vi "interface.vi"(8 "error in (no error)":errorcluster, 10 "TCP Network Connection Refnum":refnum<k5>) -> (0 "error out":errorcluster, 2 "String":string, 3 "Error Code":i32)   [LabVIEW 2017]
doc: "Reads from TCP and parses into a return string. The first four bytes of the TCP string are the error code, the next four are the length of the message. These are converted to integers and formatted at the begining of the message."
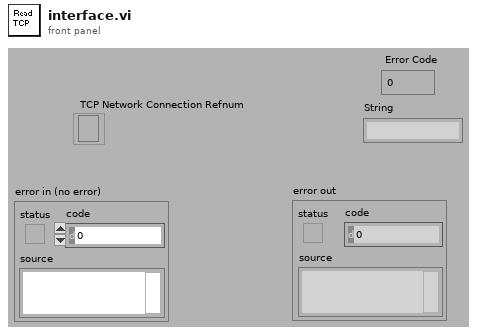
[diagram p1: front panel]
types:
  T1 = enum16{"Standard", "Buffered", "CRLF", "Immediate"}
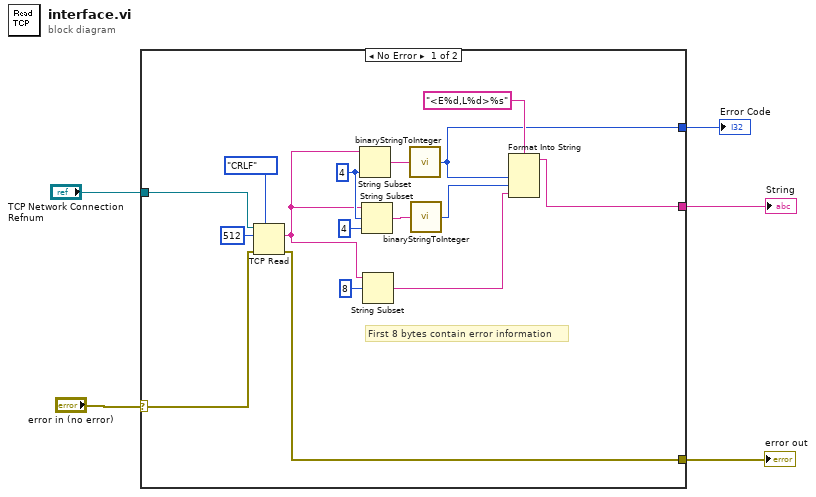
[diagram p0: block diagram]
diagram:
  n1 = case shown="No Error" "error in (no error)" {
    selector: "error in (no error)" -> [w18 w22]
    tunnel: [w17 w22] -> w4
    tunnel: [w10 _] -> w3
    tunnel: "TCP Network Connection Refnum" -> [w20 _]
    tunnel: [w6 _] -> w1
    frame No Error {
      w15 = 4 ("length (rest)")
      # "First 8 bytes contain error information"
      n2 = TCP Read(connection ID=w20, bytes to read=512, error in (no error)=w18, 7:T1."CRLF" ("mode (standard)")) -> (data out=w13:string, error out=w17:errorcluster)  [unwired: 1 in, 1 out]
      n3 = String Subset(string=w13, length (rest)=w15) -> (substring=w8:string)  [unwired: 1 in]
      n4 = String Subset(string=w13, offset (0)=w15, length (rest)=4 ("length (rest)")) -> (substring=w7:string)
      n5 = String Subset(string=w13, offset (0)=8) -> (substring=w11:string)  [unwired: 1 in]
      n6 = call "binaryStringToInteger.vi"("Binary String"=w8) -> ("Integer Output"=w6:i32)
      n7 = call "binaryStringToInteger.vi"("Binary String"=w7) -> ("Integer Output"=w9:i32)
      n8 = Format Into String(format string="<E%d,L%d>%s", w6, w9, w11) -> (resulting string=w10:string)  [unwired: 2 in, 1 out]
    }
    frame Error {
    }
  }
  "String" <- w3
  "error out" <- w4
  "Error Code" <- w1
